vi "Call DQMH Is Cloneable Module VI.vi"(8 "error in (no error)":errorcluster, 11 "DQMH Module":refnum<vi>) -> (0 "error out":errorcluster, 2 "Cloneable?":bool)   [LabVIEW 2017, in "Open DQMH Request Message Diagram.lvlib"]
uses:
  Open DQMH Request Message Diagram.lvlib
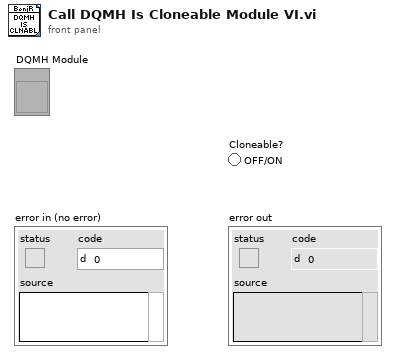
[diagram p1: front panel]
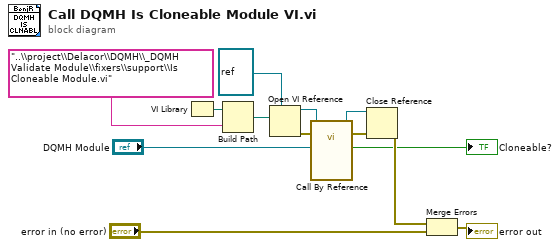
[diagram p0: block diagram]
diagram:
  n1 = VI Library() -> (path=w10:path)
  n2 = Build Path(base path=w10, name or relative path="..\\project\\Delacor\\DQMH\\_DQMH Validate Module\\fixers\\support\\Is Cloneable Module.vi") -> (appended path=w9:path)
  n3 = Open VI Reference(type specifier VI Refnum (for type only)=refnum<vi> refnum, vi path=w9) -> (vi reference=w13:refnum<vi>, error out=w6:errorcluster)  [unwired: 4 in]
  n4 = call-by-ref "?"(reference=w13, error in=w6, "DQMH Module"="DQMH Module") -> (reference out=w11:refnum<vi>, error out=w12:errorcluster, "Cloneable?"=→"Cloneable?":bool)  [unwired: 10 in]
  n5 = Close Reference(reference=w11, error in (no error)=w12) -> (error out=w8:errorcluster)
  n6 = Merge Errors(w8, "error in (no error)") -> (→"error out":errorcluster)
